vi "Gear Status FGV.vi"(8 "error in (no error)":errorcluster, 9 "Is Gear Released?":bool, 10 "Has Gear?":bool, 11 "Set? (F)":bool) -> (0 "error out":errorcluster, 2 "Is Gear Released?":bool, 3 "Has Gear?":bool)   [LabVIEW 2016, in "Intake.lvlib"]
uses:
  Intake.lvlib
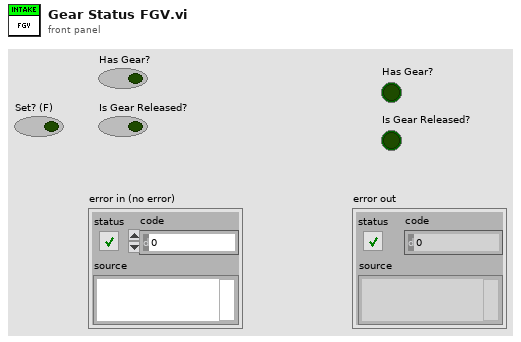
[diagram p1: front panel]
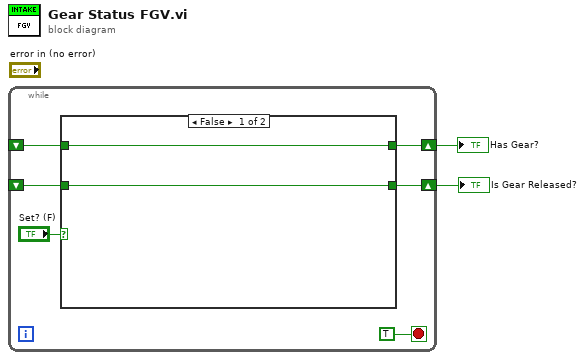
[diagram p0: block diagram]
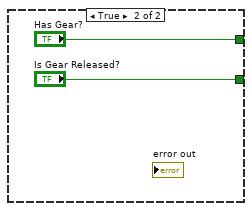
[diagram p2: hidden frame]
diagram:
  n1 = while {
    shift-right: [w4] -> w2
    shift-left: _ -> [w5]
    shift-right: [w3] -> w1
    shift-left: _ -> [w6]
    stop <- TRUE stop-if-true
    n2 = case shown="False" "Set? (F)" {
      tunnel: w6 -> [w9 _]
      tunnel: w5 -> [w10 _]
      tunnel: [w10 "Has Gear?"] -> w4
      tunnel: [w9 "Is Gear Released?"] -> w3
      frame False {
      }
      frame True {
      }
    }
  }
  "Has Gear?" <- w2
  "Is Gear Released?" <- w1
